vi "Get Msg Update Event.vi"(8 "error in (no error)":errorcluster, 11 "Comm Interface in":refnum<class "Comm Interface.lvclass">) -> (0 "error out":errorcluster, 2 "Msg Update Event":refnum<user-event>, 3 "Comm Interface out":refnum<class "Comm Interface.lvclass">)   [LabVIEW 2017, in "Comm Interface.lvlib" / "Comm Interface.lvclass"]
uses:
  Comm Interface.lvclass
  Comm Interface.lvclass/Comm Interface.ctl
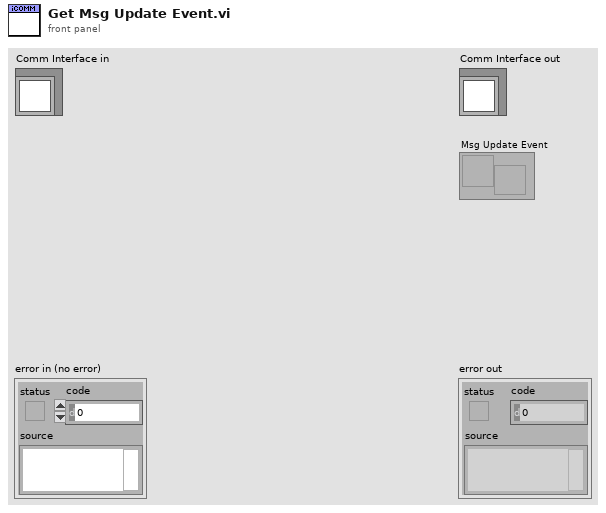
[diagram p1: front panel]
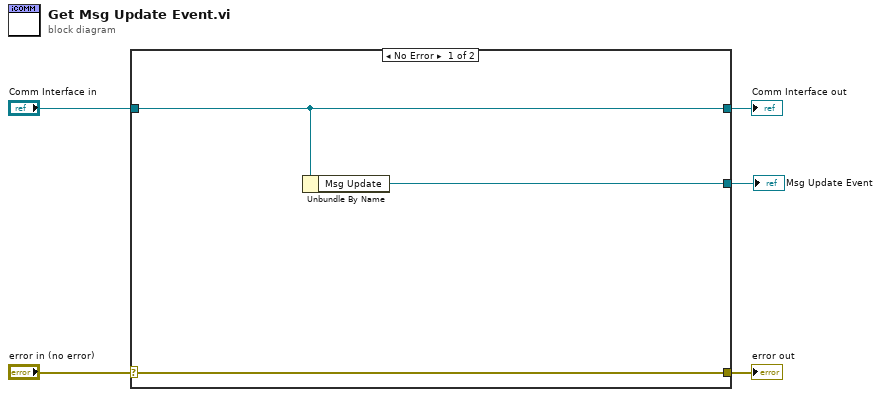
[diagram p0: block diagram]
diagram:
  n1 = case shown="No Error" "error in (no error)" {
    selector: "error in (no error)" -> [w8 w10]
    tunnel: [w8 w10] -> w4
    tunnel: [w7 w9] -> w2
    tunnel: "Comm Interface in" -> [w7 w9]
    tunnel: [w6 _] -> w1
    frame No Error {
      n2 = Unbundle By Name(w7) -> ("Msg Update"=w6:refnum<user-event>)
    }
    frame Error {
    }
  }
  "error out" <- w4
  "Comm Interface out" <- w2
  "Msg Update Event" <- w1
